vi "Build-Clear Build Folder.vi"(0 "project in":refnum<vi>, 5 "specs in":refnum<vi>[](array[refnum]), 9 "slide in":refnum<vi>, 11 "error in (no error)":errorcluster) -> (4 "project out":refnum<vi>, 6 "specs thru":refnum<vi>[](array[refnum]), 10 "slide out":refnum<vi>, 15 "error out":errorcluster)   [LabVIEW 2020]
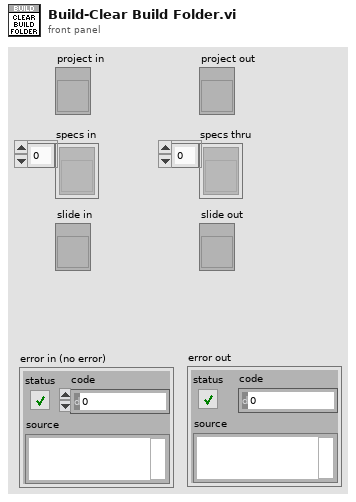
[diagram p1: front panel]
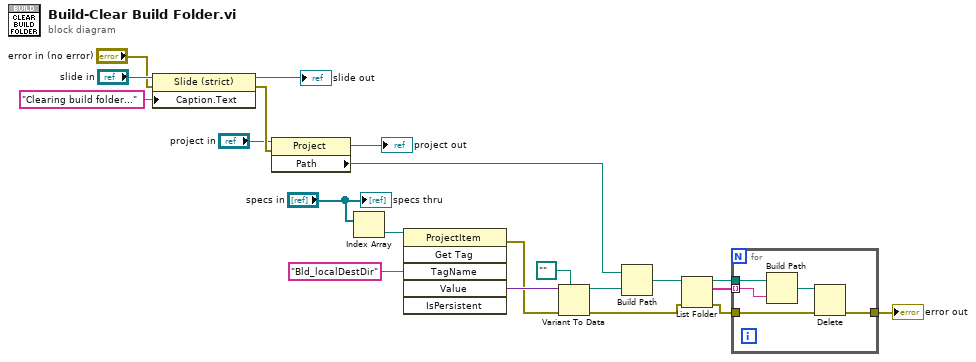
[diagram p0: block diagram]
diagram:
  n1 = property on="Property Node" class="Slide (strict)"(reference="slide in", error in="error in (no error)", "Caption.Text"="Clearing build folder...") -> (reference out=→"slide out":refnum<vi>, error out=w10:errorcluster)
  n2 = property class="Project"(reference="project in", error in=w10) -> (reference out=→"project out":refnum<vi>, "Path"=w6:path)  [unwired: 1 out]
  n3 = Index Array(array="specs in") -> (element=w18:refnum<vi>)  [unwired: 1 in]
  n4 = invoke class="ProjectItem" method="Get Tag"(reference=w18, "TagName"="Bld_localDestDir" ("Tag Name")) -> (error out=w12:errorcluster, "Value"=w14:variant)  [unwired: 4 in, 4 out]
  n5 = Variant To Data(error in=w12, type=path "", Variant=w14) -> (data=w7:path, error out=w2:errorcluster)
  n6 = Build Path(base path=w6, name or relative path=w7) -> (appended path=w5:path)
  n7 = List Folder(path=w5, error in=w2) -> (path out=w4:path, filenames=w3:string[], error out=w1:errorcluster)  [unwired: 2 in, 1 out]
  n8 = for {
    tunnel: [w26] -> w11
    tunnel: w4 -> [w25]
    tunnel: w3 -> [w24] mode=indexing
    tunnel: w1 -> [w22]
    n9 = Build Path(base path=w25, name or relative path=w24) -> (appended path=w23:path)
    n10 = Delete(path (use dialog)=w23, error in=w22) -> (error out=w26:errorcluster)  [unwired: 3 in, 2 out]
  }
  "error out" <- w11
  "specs thru" <- "specs in"
